vi "runtest Add Data to Runtest Queue.vi"(0 "Fields":T2[](array[typedef])=[{"ixField"=0, "iSequenceOrder"=0, "sxFieldId"="Serial Number", "sxSequenceId"="", "sDisplayName"="test", "sValue"="", "sUnits"="", "nDataType"=enum."timestamp", "nNextItem"=enum."Reset", "fSystem"=FALSE, "fSystemValue"=FALSE, "fRequired"=FALSE, "fSetAtTest"=FALSE, "fTestField"=FALSE, "fDeleted"=FALSE, "fIndexed"=FALSE, "fFreeList"=FALSE}, {"ixField"=0, "iSequenceOrder"=0, "sxFieldId"="Model Number", "sxSequenceId"="", "sDisplayName"="test", "sValue"="", "sUnits"="", "nDataType"=enum."timestamp", "nNextItem"=enum."Reset", "fSystem"=FALSE, "fSystemValue"=FALSE, "fRequired"=FALSE, "fSetAtTest"=FALSE, "fTestField"=FALSE, "fDeleted"=FALSE, "fIndexed"=FALSE, "fFreeList"=FALSE}], 1 "sDatasheetsCSV (\"\")":string, 2 "Test Output":T1, 3 "sTestId":string, 5 "Overwrite Existing?":bool, 7 "Print?":bool, 11 "error in (no error)":errorcluster, 12 "Test Station IP (\"\")":string, 14 "sxUsername (\"\")":string) -> (15 "error out":errorcluster)   [LabVIEW 2011]
uses:
  server/database/Fields/Field Record.ctl
  server/database/Fields/Field DataTypes.ctl
  server/database/Fields/Field NextItem.ctl
  tests/Test Output.ctl
  runtest Queue.ctl
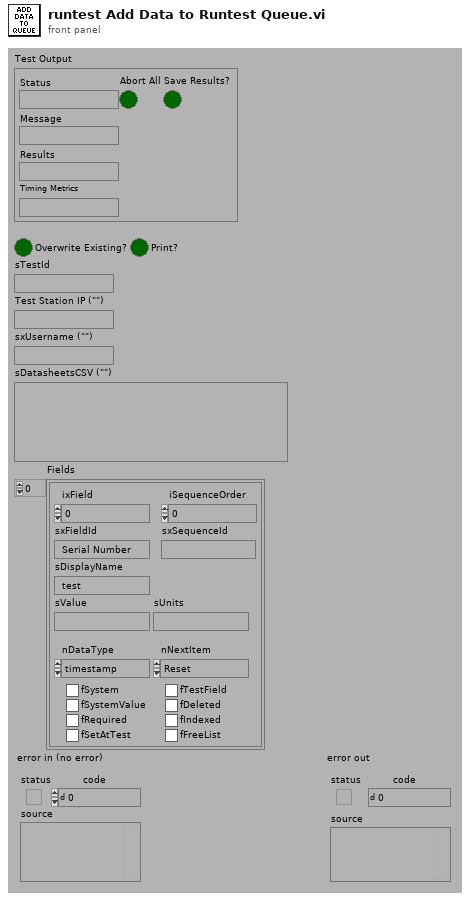
[diagram p1: front panel]
types:
  T1 = typedef "Test Output.ctl" = cluster{"Status":string, "Message":string, "Results":string, "Abort All":bool, "Save Results?":bool, "Timing Metrics":string}
  T2 = typedef "Field Record.ctl" = cluster{"ixField":i32, "iSequenceOrder":i32, "sxFieldId":string, "sxSequenceId":string, "sDisplayName":string, "sValue":string, "sUnits":string, "nDataType":T3, "nNextItem":T4, "fSystem":bool, "fSystemValue":bool, "fRequired":bool, "fSetAtTest":bool, "fTestField":bool, "fDeleted":bool, "fIndexed":bool, "fFreeList":bool}
  T3 = typedef "Field DataTypes.ctl" = enum32{"text", "numeric", "list", "timestamp", "boolean"}
  T4 = typedef "Field NextItem.ctl" = enum32{"Reset", "Retain", "Auto-Increment"}
  T5 = typedef "runtest Queue.ctl" = cluster{"Test Output":T1, "Overwrite Existing?":bool, "Print?":bool, "sTestId":string, "Test Station IP (\"\")":string, "sxUsername (\"\")":string, "sDatasheetsCSV (\"\")":string, "Fields":T2[]}
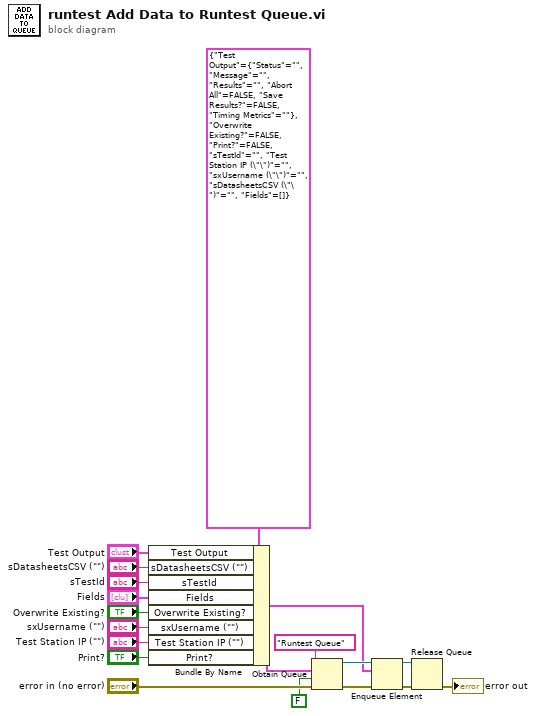
[diagram p0: block diagram]
diagram:
  n1 = Bundle By Name(cluster=T5 {"Test Output"={"Status"="", "Message"="", "Results"="", "Abort All"=FALSE, "Save Results?"=FALSE, "Timing Metrics"=""}, "Overwrite Existing?"=FALSE, "Print?"=FALSE, "sTestId"="", "Test Station IP (\"\")"="", "sxUsername (\"\")"="", "sDatasheetsCSV (\"\")"="", "Fields"=[]} ("Inputs"), "Test Output"="Test Output", "sDatasheetsCSV (\"\")"="sDatasheetsCSV (\"\")", "sTestId"="sTestId", "Fields"="Fields", "Overwrite Existing?"="Overwrite Existing?", "sxUsername (\"\")"="sxUsername (\"\")", "Test Station IP (\"\")"="Test Station IP (\"\")", "Print?"="Print?") -> (w9:T5)
  n2 = Obtain Queue(name (unnamed)="Runtest Queue", element data type=w9, create if not found? (T)=FALSE, error in (no error)="error in (no error)") -> (queue out=w10:refnum<queue>, error out=w8:errorcluster)  [unwired: 1 in, 1 out]
  n3 = Enqueue Element(queue=w10, element=w9, error in (no error)=w8) -> (queue out=w7:refnum<queue>, error out=w6:errorcluster)  [unwired: 1 in, 1 out]
  n4 = Release Queue(queue=w7, error in (no error)=w6) -> (error out=→"error out":errorcluster)  [unwired: 1 in, 2 out]
